vi "Main.vi"() -> ()   [LabVIEW 2021]
doc: "The myRIO Project template acquires acceleration data from the onboard accelerometer and displays the changes of acceleration values in a waveform chart."
uses:
  <vilib>/myRIO/Instrument Drivers/Onboard IO/I2C/typedefs/I2C User Configuration.ctl
  <vilib>/myRIO/Instrument Drivers/Onboard IO/I2C/typedefs/I2C Transfer Rate.ctl
  <vilib>/Platform/TimedLoop/XDataNode/timing_clust.ctl
  <vilib>/Platform/TimedLoop/XDataNode/nitl_modes.ctl
  <vilib>/Platform/TimedLoop/XDataNode/wakeup.ctl
  <vilib>/myRIO/Common/Instrument Driver Framework/myRIO v1.0/UART/vis/myRIO v1.0 Close UART.vi
  <vilib>/Utility/error.llb/Error Cluster From Error Code.vi
  <vilib>/myRIO/Common/Instrument Driver Framework/myRIO v1.0/I2C/vis/myRIO v1.0 Configure I2C.vi
  <vilib>/myRIO/Common/Instrument Driver Framework/myRIO v1.0/DIO/vis/myRIO v1.0 Read DIO.vi
  <vilib>/myRIO/Common/Instrument Driver Framework/myRIO v1.0/I2C/vis/myRIO v1.0 Write I2C.vi
  <vilib>/myRIO/Common/Instrument Driver Framework/myRIO v1.0/AI/vis/myRIO v1.0 Read AI.vi
  <vilib>/express/express analysis/Spectral/Block/exnSpectralBlock spectral measurements power poly.vi
  <vilib>/express/express analysis/Spectral/Block/exnSpectralBlock spectral measurements power DDT.vi
  <vilib>/myRIO/Common/Instrument Driver Framework/Utilities/vis/FPGA Ref Manager.vi
  <vilib>/myRIO/Common/Instrument Driver Framework/myRIO v1.0/myRIO v1.0 Reset FPGA.vi
  <vilib>/myRIO/Common/Instrument Driver Framework/myRIO v1.0/IRQ/vis/myRIO v1.0 IRQ Info FGV.vi
  <vilib>/myRIO/Common/Instrument Driver Framework/myRIO v1.0/IRQ/vis/myRIO v1.0 Timer IRQ Info FGV.vi
  <vilib>/myRIO/Common/Instrument Driver Framework/myRIO v1.0/IRQ/vis/myRIO v1.0 ISR Agent.vi
  <vilib>/myRIO/Instrument Drivers/Utilities/vis/Reset Index.vi
  <vilib>/myRIO/Common/Instrument Driver Framework/myRIO v1.0/Resource Manager/vis/myRIO v1.0 Block Write Resource Manager.vi
  <vilib>/Platform/TimedLoop/XDataNode/XDataNode.xnode
  <vilib>/express/express analysis/Spectral/XNode/ExpressSpectralMeasurementsBlockNode.xnode
  <vilib>/Platform/TimedLoop/XDataNode/XDNodeRunTimeDep.lvlib
  <vilib>/myRIO/Instrument Drivers/Onboard IO/AI/AI.lvlib
  <vilib>/myRIO/Instrument Drivers/Onboard IO/DIO/DIO.lvlib
  <vilib>/Analysis/NI_AAL_SigProc.lvlib
  <vilib>/Analysis/NI_AALPro.lvlib
  <vilib>/myRIO/Instrument Drivers/Utilities/Utilities.lvlib
  <vilib>/myRIO/Instrument Drivers/Onboard IO/I2C/I2C.lvlib
panel:
  in  "Stop Button 2":bool
  in  "Tab Control":T1(tab)
  out "SpO2 (%)":dbl
  in  "Collect Data 3":bool
  in  "R Offset":dbl=0.6
  in  "IR Offset":dbl=0.24
  in  "% Threshold":dbl=0.5 format="%0.2f"
  in  "Width":i32=20 min=3
  out "Heart Rate (bpm)":i32
  out "Filtered Readings 2":dynamicdata(graph)
  out "Frequency Analysis Power Spectrum":dynamicdata(graph)
  in  "Period (> 3s)":dbl=10.0
  in  "Interval (ms)":i64=1
  in  "[ESC] 3":bool
  out "LCD display":string
  out "Imax R":dbl
  out "Imin R":dbl
  out "Imax IR":dbl
  out "Imin IR":dbl
  out "Max Freq R":dbl
  out "Max Freq IR":dbl
  in  "dt (ms)":i64=1
  out "Vpp R":dbl format="%.2p"
  out "Vpp IR":dbl format="%.2p"
  in  "Period (s)":dbl=10.0
  in  "Collect Data 2":bool
  out "Power Spectrum":dynamicdata(graph)
  out "Filtered Readings":dynamicdata(graph)
  out "Heart Rate (bpm)":i32
  in  "width":i32=20 min=3
  in  "threshold":dbl=0.002 format="%0.4f"
  in  "R Offset":dbl
  in  "IR Offset":dbl
  out "Channel Readings":T2(graph)
  in  "[ESC] 2":bool
  out "Blood Oxygen Saturation":dbl
  in  "Absorbance Ratio (R / IR)":dbl(slide) scale=0.0..1.0
  in  "Use Direct Input":bool
  out "LCD display":string
  in  "[ESC]":bool
  in  "Blood Oxygen Input":dbl
  in  "Heart Rate":i32
  in  "Display Data":bool
  in  "eHb, lam1":dbl=0.81
  in  "eHb, lam2":dbl=0.18
  in  "eHbO2, lam1":dbl=0.08
  in  "eHbO2, lam2":dbl=0.29
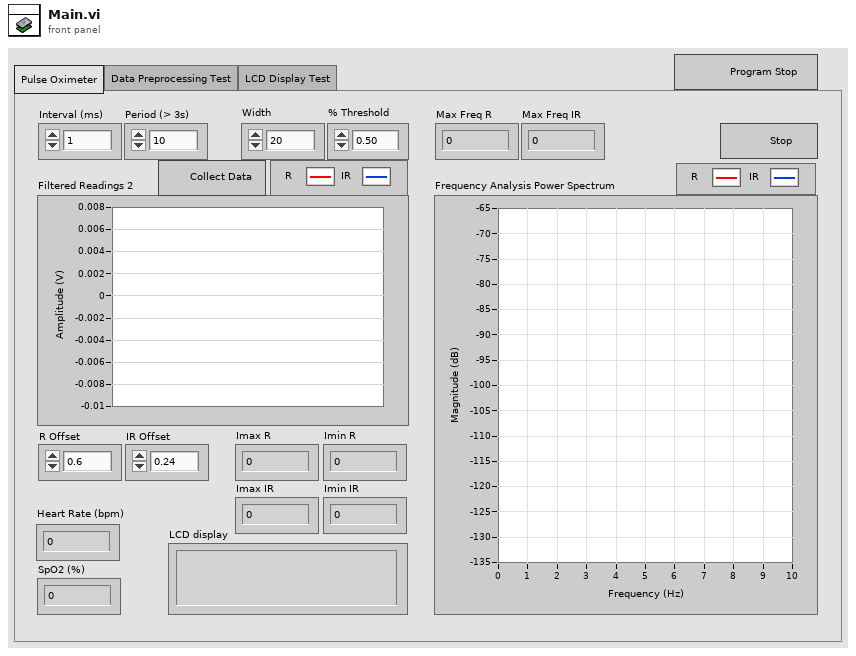
[diagram p1: front panel]
types:
  T1 = enum32{"Pulse Oximeter", "Data Preprocessing Test", "LCD Display Test", "Custom Graphs"}
  T2 = cluster{"dbl Scaled Value":dbl, "dbl Scaled Value":dbl}
  T3 = typedef "I2C.lvlib/I2C User Configuration.ctl" = cluster{"I2C Transfer Rate":T4}
  T4 = typedef "I2C.lvlib/I2C Transfer Rate.ctl" = enum16{"Standard mode (100 kbps)", "Fast mode (400 kbps)"}
  T5 = typedef "I2C.lvlib/I2C Reference.ctl" = cluster{"myRIO Reference":T6, "I2C Channels Enum":T10, "I2C Configuration":T11}
  T6 = typedef "myRIO Generic Hardware Reference.ctl" = cluster{"myRIO Model":T7, "myRIO Hardware Reference":T8}
  T7 = typedef "Hardware Version Enum.ctl" = enum16{"Unknown", "myRIO-1900", "myRIO-1950", "roboRIO", "NI ELVIS RIO CM", "ELVIS III"}
  T8 = typedef "myRIO v1.0 Reference.ctl" = cluster{"Generic FPGA Reference":T9, "Allow multiple opens":bool}
  T9 = typedef "Generic FPGA Reference.ctl" = refnum<k20>
  T10 = typedef "I2C Channels Enum.ctl" = enum16{"Not Connected", "A/I2C", "B/I2C", "I2C/I2C"}
  T11 = typedef "I2C.lvlib/I2C Configuration.ctl" = cluster{"I2C Transfer Rate":T4}
  T12 = typedef "DIO.lvlib/DIO Reference.ctl" = cluster{"myRIO Reference":T6, "DIO Channels List":T13}
  T13 = typedef "DIO Channels List.ctl" = T14[]
  T14 = typedef "DIO Channels Enum.ctl" = enum16{"Not Connected", "C/DIO0", "C/DIO1", "C/DIO2", "C/DIO3", "C/DIO4", "C/DIO5", "C/DIO6", "C/DIO7", "A/DIO0", "A/DIO1", "A/DIO2", "A/DIO3", "A/DIO4", "A/DIO5", "A/DIO6", "A/DIO7", "A/DIO8", "A/DIO9", "A/DIO10", "A/DIO11", "A/DIO12", "A/DIO13", "A/DIO14", "A/DIO15", "A/DIO16", "A/DIO17", "A/DIO18", "A/DIO19", "B/DIO0", "B/DIO1", "B/DIO2", "B/DIO3", "B/DIO4", "B/DIO5", "B/DIO6", "B/DIO7", "B/DIO8", "B/DIO9", "B/DIO10", "B/DIO11", "B/DIO12", "B/DIO13", "B/DIO14", "B/DIO15", "B/DIO16", "B/DIO17", "B/DIO18", "B/DIO19", "LED0", "LED1", "LED2", "LED3", "Button0", "DIO/DIO0", "DIO/DIO1", "DIO/DIO2", "DIO/DIO3", "DIO/DIO4", "DIO/DIO5", "DIO/DIO6", "DIO/DIO7", "DIO/DIO8", "DIO/DIO9", "SPI/CS0", "SPI/CS1", "SPI/CS2", "SPI/CS3", "LED RADIO (Green)", "LED RADIO (Red)", "LED COMM (Green)", "LED COMM (Red)", "LED MODE (Green)", "LED MODE (Red)"}
  T15 = typedef "AI.lvlib/AI Reference.ctl" = cluster{"myRIO Reference":T6, "AI Channels List":T16, "AI Scaling Constants List":T18}
  T16 = typedef "AI Channels List.ctl" = T17[]
  T17 = typedef "AI Channels Enum.ctl" = enum16{"Not Connected", "AudioIn/Left", "AudioIn/Right", "C/AI0", "C/AI1", "A/AI0", "A/AI1", "A/AI2", "A/AI3", "A/AI4", "A/AI5", "A/AI6", "A/AI7", "B/AI0", "B/AI1", "B/AI2", "B/AI3", "B/AI4", "B/AI5", "B/AI6", "B/AI7", "AI/AI0", "AI/AI1", "AI/AI2", "AI/AI3", "A/AI0 (DIFF)", "A/AI1 (DIFF)", "A/AI2 (DIFF)", "A/AI3 (DIFF)", "B/AI0 (DIFF)", "B/AI1 (DIFF)", "B/AI2 (DIFF)", "B/AI3 (DIFF)"}
  T18 = typedef "Analog Scaling Constants List.ctl" = T19[]
  T19 = typedef "Analog Scaling Constants.ctl" = cluster{"LSB Weight (Volts)":dbl, "Offset (Volts)":dbl, "Signed?":bool}
  T20 = typedef "XDNodeRunTimeDep.lvlib/timing_clust.ctl" = cluster{"Expected End [f-1]":u64, "Actual End [f-1]":u64, "Finished Late? [f-1]":bool, "Expected End [i-1]":u64, "Actual End [i-1]":u64, "Finished Late? [i-1]":bool, "Expected Start [i]":u64, "Actual Start [i]":u64, "Expected Start [f]":u64, "Actual Start [f]":u64, "Source Name":string, "Structure Name":string, "Period":i64, "Deadline":i64, "Offset":i64, "Start":i64, "Priority":i32, "Timeout":i32, "Mode":T21, "Wakeup Reason":T22, "Error":errorcluster, "Source Type":string, "Secondary Source Type":string, "Global End Time":u64, "Global Start Time":u64, "Frame Duration":u64, "Iteration Duration":u64, "Assigned CPU":i32, "I/O Scan Engine Mode":u32}
  T21 = typedef "XDNodeRunTimeDep.lvlib/nitl_modes.ctl" = enum32{"No Change", "Process missed periods, maintain original phase", "Discard missed periods, maintain original phase", "Process missed periods, ignore original phase", "Discard missed periods, ignore original phase"}
  T22 = typedef "XDNodeRunTimeDep.lvlib/wakeup.ctl" = enum32{"Normal", "Aborted", "Asynchronous wakeup", "Timing source error", "Timed loop error", "Timeout"}
  T23 = cluster{"averaging mode":u16, "weighting mode":u16, "number of averages":u32}
  T24 = cluster{"dB On (F)":bool, "unwrap phase (F)":bool, "convert to degree (F)":bool}
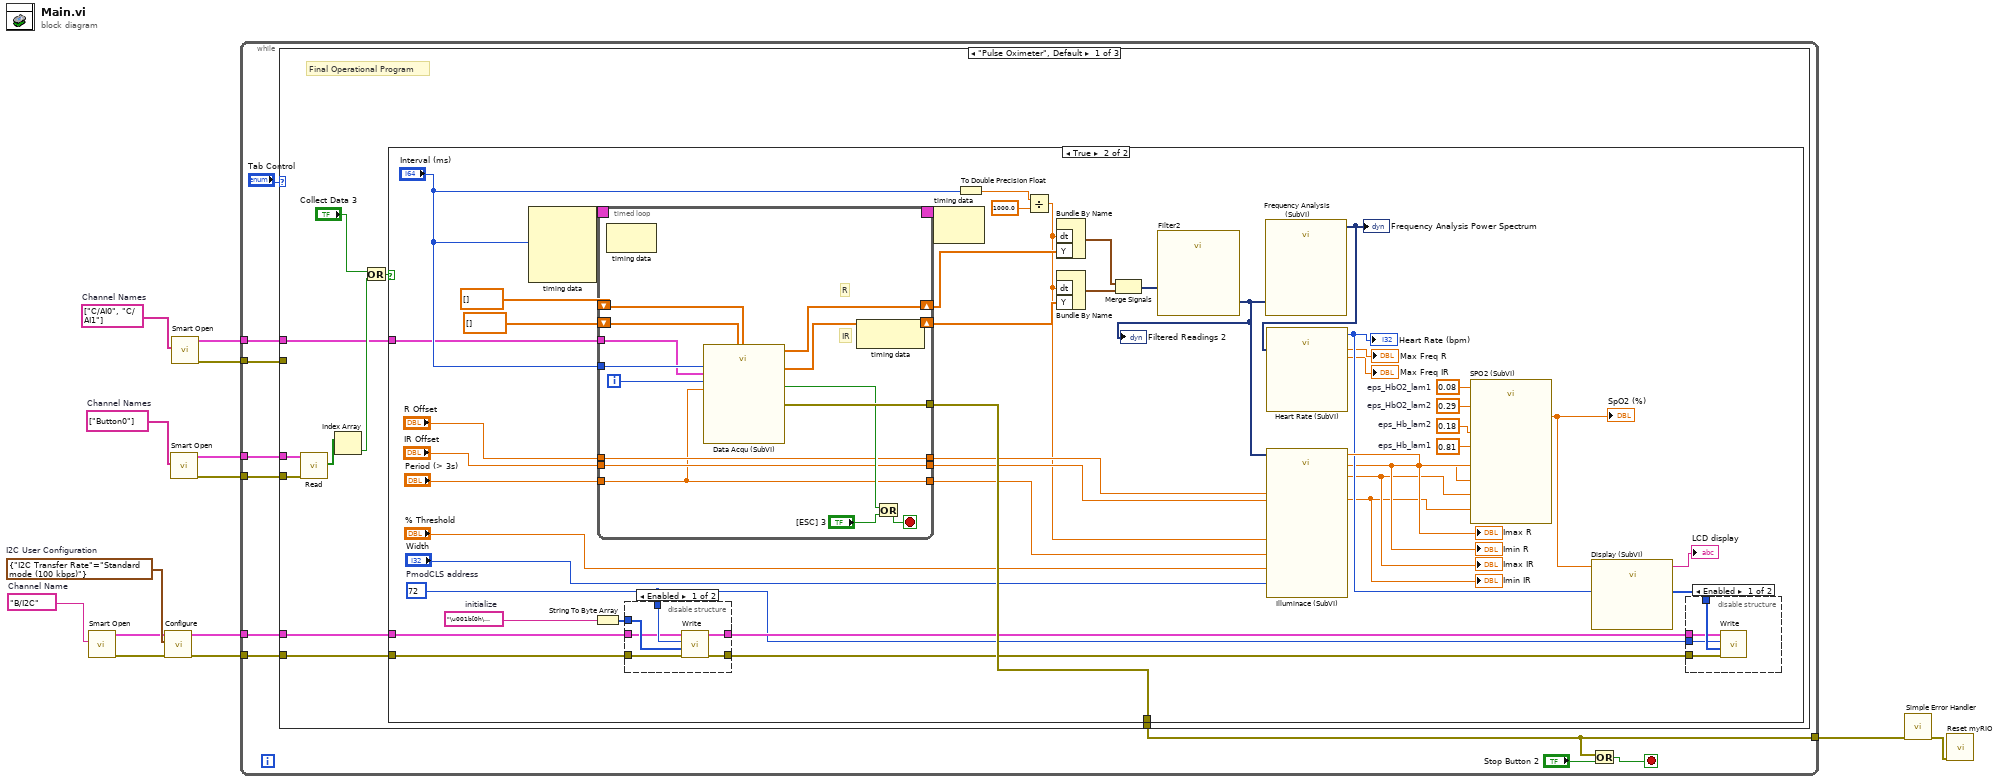
[diagram p0: block diagram]
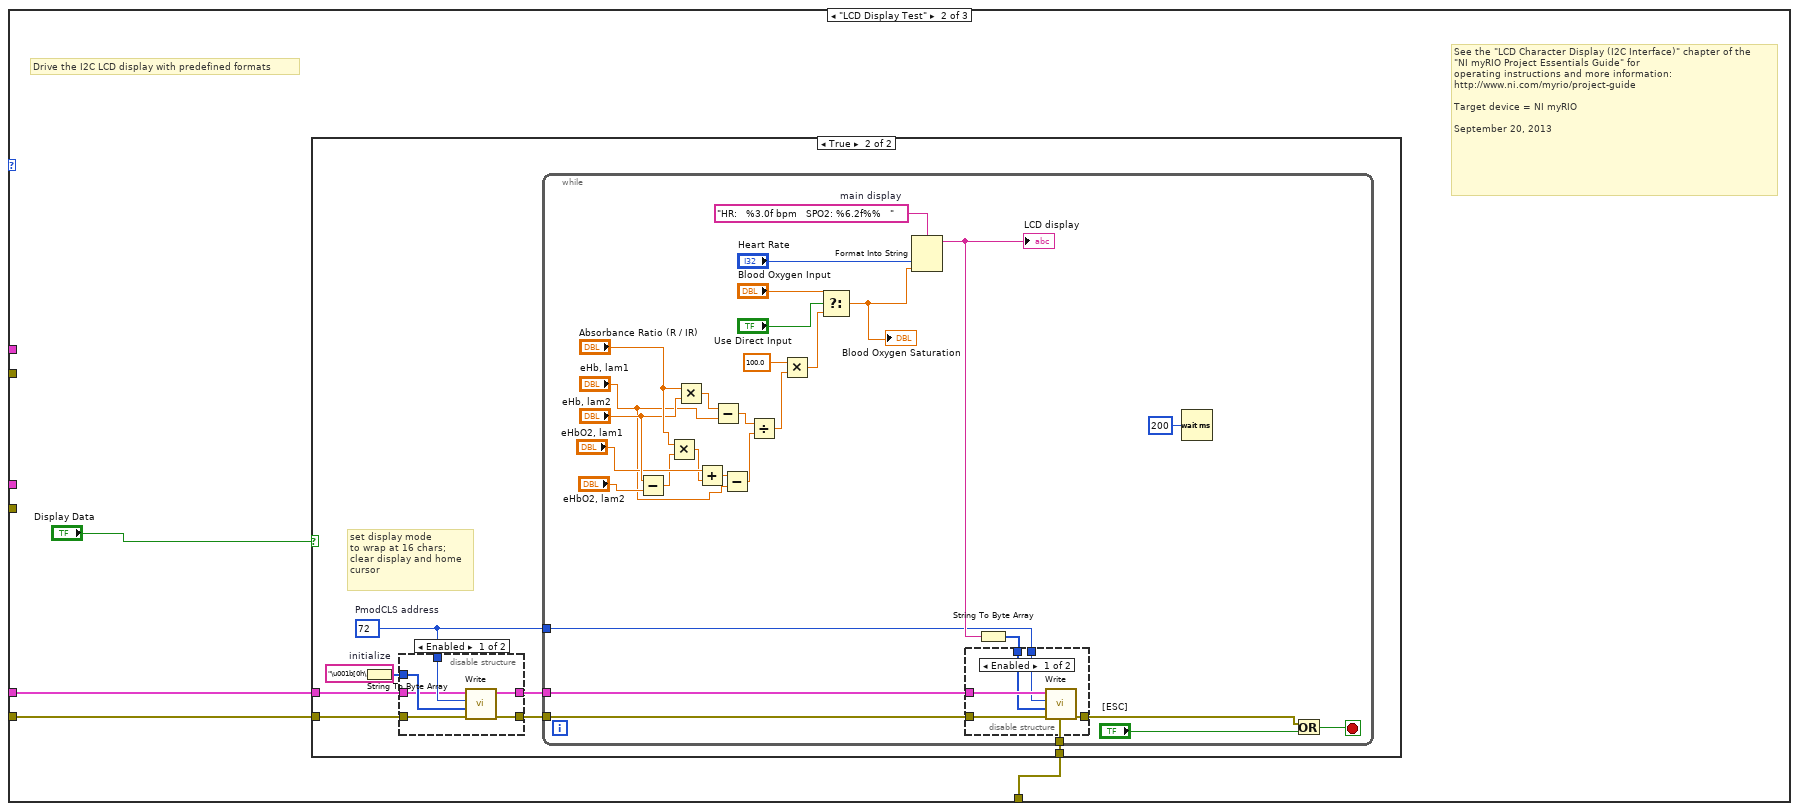
[diagram p5: hidden frame]
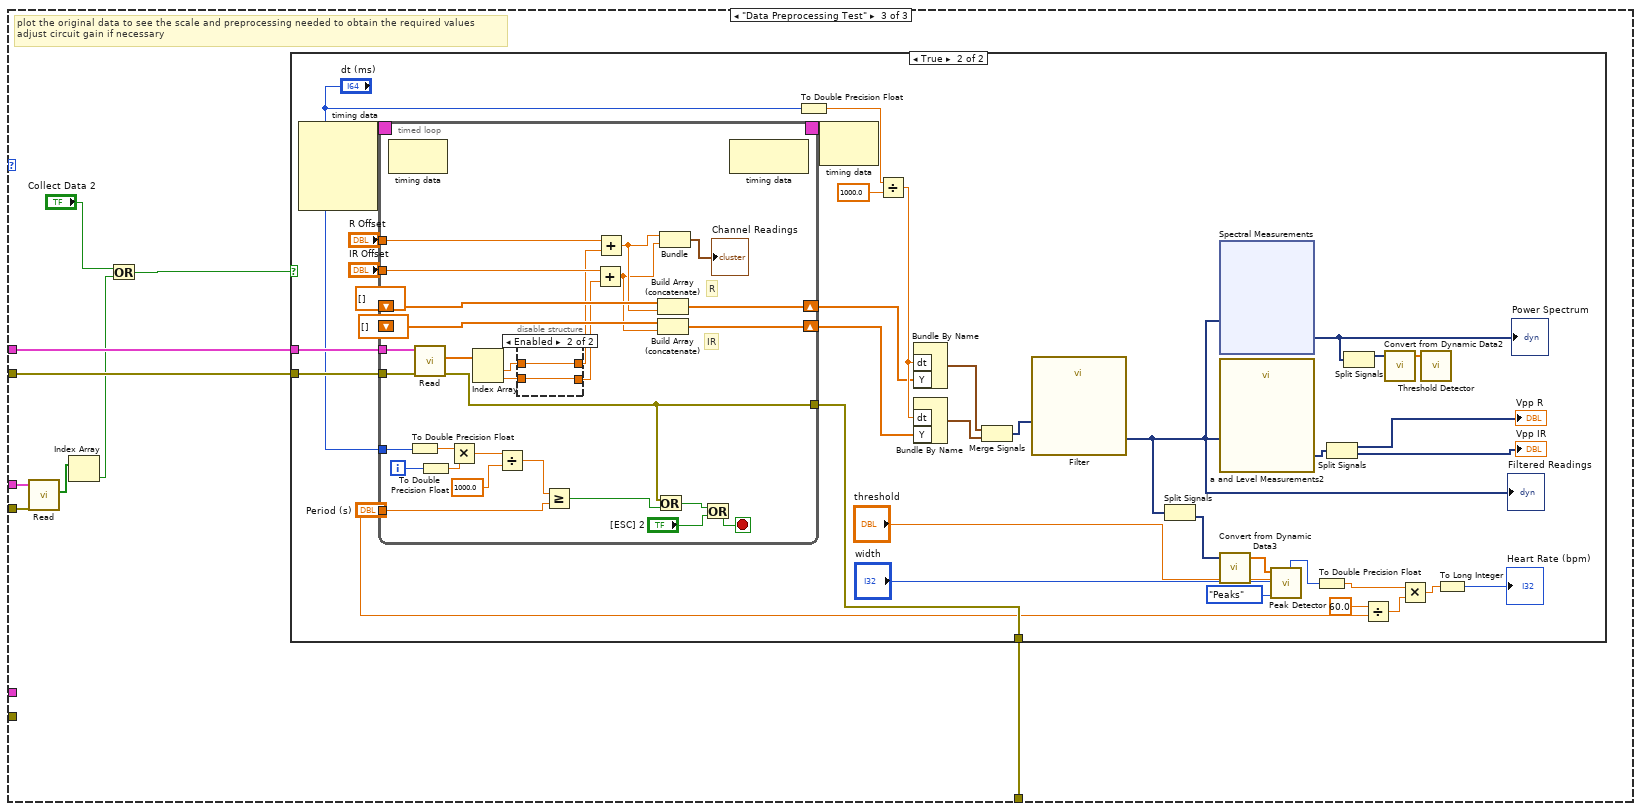
[diagram p9: hidden frame]
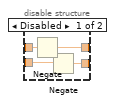
[diagram p11: hidden frame]
diagram:
  w5 = T3 {"I2C Transfer Rate"=enum."Standard mode (100 kbps)"}  # I2C User Configuration
  w6 = tag "B/I2C"  # Channel Name
  w11 = tag[] ["Button0"]  # Channel Names
  w14 = tag[] ["C/AI0", "C/AI1"]  # Channel Names
  n1 = call <vilib>:"Smart Open.vi"("Channel Name"=w6) -> ("error out"=w3:errorcluster, "I2C Ref Out"=w4:T5)  [unwired: 9 in]
  n2 = call <vilib>:"Configure.vi"("error in (no error)"=w3, "I2C User Configuration"=w5, "I2C Ref In"=w4) -> ("error out"=w2:errorcluster, "I2C Ref Out"=w1:T5)  [unwired: 7 in]
  n3 = call <vilib>:"Smart Open.vi"("Channel Names"=w11) -> ("error out"=w9:errorcluster, "DIO Ref Out"=w10:T12)  [unwired: 9 in]
  n4 = call <vilib>:"Smart Open.vi"("Channel Names"=w14) -> ("error out"=w12:errorcluster, "AI Ref Out"=w13:T15)  [unwired: 9 in]
  n5 = while {
    tunnel: w13 -> [w24]
    tunnel: w12 -> [w23]
    tunnel: w10 -> [w21]
    tunnel: w9 -> [w20]
    tunnel: [w17] -> w7
    tunnel: w2 -> [w15]
    tunnel: w1 -> [w16]
    stop <- w18 stop-if-true
    n6 = case shown="\"Pulse Oximeter\", Default" "Tab Control" {
      tunnel: w24 -> [w27 _ w176]
      tunnel: w23 -> [_ _ w175]
      tunnel: w21 -> [w31 _ w174]
      tunnel: w20 -> [w30 _ w173]
      tunnel: [w28 w117 w168] -> w17
      tunnel: w16 -> [w26 w115 _]
      tunnel: w15 -> [w25 w114 _]
      frame "Pulse Oximeter", Default {
        # "Final Operational Program"
        n7 = call <vilib>:"Read.vi"("error in (no error)"=w30, "DIO Ref In"=w31) -> ("Values"=w34:bool[])  [unwired: 7 in, 2 out]
        n8 = Index Array(array=w34) -> (element=w32:bool)  [unwired: 1 in]
        n9 = Or(x="Collect Data 3", y=w32) -> (x .or. y?=w29:bool)
        n10 = case shown="True" w29 {
          tunnel: [_ w68] -> w28
          tunnel: w27 -> [_ w62]
          tunnel: w26 -> [_ w45]
          tunnel: w25 -> [_ w44]
          frame False {
          }
          frame True {
            w46 = u8 72  # PmodCLS address
            w50 = "\u001b[0h\u001b[j"  # initialize
            w63 = 0.81  # eps_Hb_lam1
            w65 = 0.29  # eps_HbO2_lam2
            w67 = 0.08  # eps_HbO2_lam1
            w64 = 0.18  # eps_Hb_lam2
            n11 = node-c288("Interval (ms)") -> (w80:T20)  [unwired: 3 in]
            n12 = String To Byte Array(string=w50) -> (unsigned byte array=w49:u8[])
            n13 = timed-loop {
              timing: w80 -> [_]
              timing-out: [_] -> w79
              shift-right: [w94] -> w40
              shift-left: dbl[] [] -> [w93]
              shift-right: [w92] -> w39
              shift-left: dbl[] [] -> [w91]
              tunnel: "Interval (ms)" -> [w85]
              tunnel: "Period (> 3s)" -> [w81]
              tunnel: "R Offset" -> [w82]
              tunnel: "IR Offset" -> [w83]
              tunnel: [w89] -> w68
              tunnel: w62 -> [w84]
              tunnel: [w83] -> w37
              tunnel: [w82] -> w38
              tunnel: [w81] -> w35
              i -> [w90]
              stop <- w88 stop-if-true
              # "IR"
              # "R"
              n14 = node-c288() -> ()  [unwired: 1 in, 1 out]
              n15 = call "Data Acqu (SubVI).vi"("Period (s) in"=w81, "Numeric"=w90, "AI Ref In"=w84, "dt (ms) in"=w85, "Array in"=w91, "Array 3"=w93) -> ("error out"=w89:errorcluster, "Boolean"=w87:bool, "Array out"=w92:dbl[], "Array 4"=w94:dbl[])  [unwired: 2 in]
              n16 = node-c288() -> ()  [unwired: 1 in, 1 out]
              n17 = Or(x=w87, y="[ESC] 3") -> (x .or. y?=w88:bool)
            }
            n18 = disable-structure shown="Enabled" {
              disable-tunnel: w46 -> [w105 _]
              disable-tunnel: w44 -> [w100 w106]
              disable-tunnel: w49 -> [w104 _]
              disable-tunnel: w45 -> [w101 w107]
              disable-tunnel: [w103 w106] -> w47
              disable-tunnel: [w102 w107] -> w48
              frame Enabled {
                n19 = call <vilib>:"Write.vi"("error in (no error)"=w100, "Bytes to Write"=w104, "Slave Address (7-bit)"=w105, "I2C Ref In"=w101) -> ("error out"=w103:errorcluster, "I2C Ref Out"=w102:T5)  [unwired: 6 in]
              }
              frame Disabled {
              }
            }
            n20 = node-c288(w79) -> ()  [unwired: 1 out]
            n21 = To Double Precision Float(number="Interval (ms)") -> (double precision float=w77:dbl)
            n22 = Divide(x=w77, y=1000.0) -> (x/y=w36:dbl)
            n23 = Bundle By Name("dt"=w36, "Y"=w40) -> (w74:waveform(dbl))  [unwired: 1 in]
            n24 = Bundle By Name("dt"=w36, "Y"=w39) -> (w73:waveform(dbl))  [unwired: 1 in]
            n25 = Merge Signals(w74, w73) -> (w72:dynamicdata)
            n26 = call "Filter2"("Signal"=w72) -> ("Filtered Signal"=w61:dynamicdata)  [unwired: 9 in, 1 out]
            "Filtered Readings 2" <- w61
            n27 = call "Frequency Analysis (SubVI).vi"("Filtered Signal"=w61) -> ("Power Spectrum"=w41:dynamicdata)  [unwired: 8 in, 2 out]
            "Frequency Analysis Power Spectrum" <- w41
            n28 = call "Heart Rate (SubVI).vi"("Power Spectrum"=w41) -> ("Max Freq IR"=→"Max Freq IR":dbl, "Max Freq R"=→"Max Freq R":dbl, "Avg HR bpm"=w56:i32)  [unwired: 7 in, 1 out]
            "Heart Rate (bpm)" <- w56
            n29 = call "Illuminace (SubVI).vi"("R Offset"=w38, "Interval"=w36, "IR Offset"=w37, "Period (> 3s)"=w35, "Width"="Width", "% Threshold"="% Threshold", "Filtered Signal"=w61) -> ("Imax IR"=w53:dbl, "Imin R"=w54:dbl, "Imax R"=w58:dbl, "Imin IR"=w52:dbl)  [unwired: 1 out]
            "Imax R" <- w58
            "Imin R" <- w54
            "Imax IR" <- w53
            "Imin IR" <- w52
            n30 = call "SPO2 (SubVI).vi"("I_max_lam1"=w58, "eps_Hb_lam2"=w64, "I_min_lam2"=w52, "eps_Hb_lam1"=w63, "I_max_lam2"=w53, "eps_HbO2_lam2"=w65, "I_min_lam1"=w54, "eps_HbO2_lam1"=w67) -> ("Numeric"=w55:dbl)  [unwired: 3 in]
            "SpO2 (%)" <- w55
            n31 = call "Display (SubVI).vi"("Numeric 2"=w56, "Numeric"=w55) -> ("Formatted Array"=w51:u8[], "Formatted String"=→"LCD display":string)  [unwired: 8 in]
            n32 = disable-structure shown="Enabled" {
              disable-tunnel: w47 -> [w108 w112]
              disable-tunnel: w51 -> [w111 _]
              disable-tunnel: w46 -> [w110 _]
              disable-tunnel: w48 -> [w109 _]
              frame Enabled {
                n33 = call <vilib>:"Write.vi"("error in (no error)"=w108, "Bytes to Write"=w111, "Slave Address (7-bit)"=w110, "I2C Ref In"=w109) -> ()  [unwired: 6 in, 2 out]
              }
              frame Disabled {
              }
            }
          }
        }
      }
      frame "LCD Display Test" {
        # "See the \"LCD Character Display (I2C Interface)\" chapter of the\n\"NI myRIO Project Essentials Guide\" for\noperating instructions and more information: \nhttp://www.ni.com/myrio/project-guide\n\nTarget device = NI myRIO\n\nSeptember 20, 2013"
        # "Drive the I2C LCD display with predefined formats"
        n34 = case shown="True" "Display Data" {
          tunnel: [_ w124] -> w117
          tunnel: w115 -> [_ w119]
          tunnel: w114 -> [_ w118]
          frame False {
          }
          frame True {
            w123 = u8 72  # PmodCLS address
            w125 = "\u001b[0h\u001b[j"  # initialize
            # "set display mode\nto wrap at 16 chars;\nclear display and home\ncursor"
            n35 = String To Byte Array(string=w125) -> (unsigned byte array=w122:u8[])
            n36 = disable-structure shown="Enabled" {
              disable-tunnel: w123 -> [w131 _]
              disable-tunnel: w118 -> [w126 w132]
              disable-tunnel: w122 -> [w130 _]
              disable-tunnel: w119 -> [w127 w133]
              disable-tunnel: [w129 w132] -> w121
              disable-tunnel: [w128 w133] -> w120
              frame Enabled {
                n37 = call <vilib>:"Write.vi"("error in (no error)"=w126, "Bytes to Write"=w130, "Slave Address (7-bit)"=w131, "I2C Ref In"=w127) -> ("error out"=w129:errorcluster, "I2C Ref Out"=w128:T5)  [unwired: 6 in]
              }
              frame Disabled {
              }
            }
            n38 = while {
              tunnel: w123 -> [w152]
              tunnel: [w155] -> w124
              tunnel: w121 -> [w156]
              tunnel: w120 -> [w154]
              stop <- w159 stop-if-true
              w161 = "HR:   %3.0f bpm   SPO2: %6.2f%%   "  # main display
              n39 = Subtract(x="eHb, lam2", y="eHbO2, lam2") -> (x-y=w140:dbl)
              n40 = Multiply(x="Absorbance Ratio (R / IR)", y=w140) -> (x*y=w139:dbl)
              n41 = Multiply(x="Absorbance Ratio (R / IR)", y="eHb, lam2") -> (x*y=w148:dbl)
              n42 = Add(x="eHbO2, lam1", y=w139) -> (x+y=w142:dbl)
              n43 = Subtract(x=w148, y="eHb, lam1") -> (x-y=w147:dbl)
              n44 = Subtract(x=w142, y="eHb, lam1") -> (x-y=w138:dbl)
              n45 = Divide(x=w147, y=w138) -> (x/y=w137:dbl)
              n46 = Multiply(x=100.0, y=w137) -> (x*y=w135:dbl)
              n47 = Select(t="Blood Oxygen Input", s="Use Direct Input", f=w135) -> (s? t:f=w134:dbl)
              "Blood Oxygen Saturation" <- w134
              n48 = Format Into String "Format Into String"(format string=w161, "Heart Rate", w134) -> (resulting string=w157:string)  [unwired: 2 in, 1 out]
              "LCD display" <- w157
              n49 = String To Byte Array(string=w157) -> (unsigned byte array=w153:u8[])
              n50 = disable-structure shown="Enabled" {
                disable-tunnel: w156 -> [w166 w167]
                disable-tunnel: [w165 w167] -> w155
                disable-tunnel: w154 -> [w164 _]
                disable-tunnel: w153 -> [w163 _]
                disable-tunnel: w152 -> [w162 _]
                frame Enabled {
                  n51 = call <vilib>:"Write.vi"("error in (no error)"=w166, "Bytes to Write"=w163, "Slave Address (7-bit)"=w162, "I2C Ref In"=w164) -> ("error out"=w165:errorcluster)  [unwired: 6 in, 1 out]
                }
                frame Disabled {
                }
              }
              n52 = Wait (ms)(milliseconds to wait=u32 200) -> ()  [unwired: 1 out]
              n53 = Or(x=w155, y="[ESC]") -> (x .or. y?=w159:bool)
            }
          }
        }
      }
      frame "Data Preprocessing Test" {
        # "plot the original data to see the scale and preprocessing needed to obtain the required values\nadjust circuit gain if necessary"
        n54 = call <vilib>:"Read.vi"("error in (no error)"=w173, "DIO Ref In"=w174) -> ("Values"=w172:bool[])  [unwired: 7 in, 2 out]
        n55 = Index Array(array=w172) -> (element=w169:bool)  [unwired: 1 in]
        n56 = Or(x="Collect Data 2", y=w169) -> (x .or. y?=w170:bool)
        n57 = case shown="True" w170 {
          tunnel: w176 -> [_ w211]
          tunnel: w175 -> [_ w210]
          tunnel: [_ w181] -> w168
          frame False {
          }
          frame True {
            n58 = node-c288("dt (ms)") -> (w213:T20)  [unwired: 3 in]
            n59 = timed-loop {
              timing: w213 -> [_]
              timing-out: [_] -> w212
              tunnel: w211 -> [w242]
              tunnel: w210 -> [w241]
              shift-right: [w240] -> w205
              shift-left: dbl[] [] -> [w239]
              shift-right: [w238] -> w204
              shift-left: dbl[] [] -> [w237]
              tunnel: "dt (ms)" -> [w232]
              tunnel: "Period (s)" -> [w229]
              tunnel: "R Offset" -> [w227]
              tunnel: "IR Offset" -> [w226]
              tunnel: [w221] -> w181
              i -> [w234]
              stop <- w220 stop-if-true
              # "IR"
              # "R"
              n60 = node-c288() -> ()  [unwired: 1 in, 1 out]
              n61 = To Double Precision Float(number=w232) -> (double precision float=w231:dbl)
              n62 = call <vilib>:"Read.vi"("error in (no error)"=w241, "AI Ref In"=w242) -> ("error out"=w221:errorcluster, "Values"=w228:dbl[])  [unwired: 7 in, 1 out]
              n63 = To Double Precision Float(number=w234) -> (double precision float=w233:dbl)
              n64 = Multiply(x=w231, y=w233) -> (x*y=w236:dbl)
              n65 = Index Array(array=w228) -> (element #1=w217:dbl, element #2=w215:dbl)  [unwired: 2 in]
              n66 = Divide(x=w236, y=1000.0) -> (x/y=w230:dbl)
              n67 = disable-structure shown="Enabled" {
                disable-tunnel: w217 -> [w246 w248]
                disable-tunnel: [w245 w248] -> w216
                disable-tunnel: w215 -> [w244 w247]
                disable-tunnel: [w243 w247] -> w214
                frame Disabled {
                  n68 = Negate(x=w246) -> (-x=w245:dbl)
                  n69 = Negate(x=w244) -> (-x=w243:dbl)
                }
                frame Enabled {
                }
              }
              n70 = Greater Or Equal?(x=w230, y=w229) -> (x >= y?=w222:bool)
              n71 = Add(x=w226, y=w214) -> (x+y=w223:dbl)
              n72 = Add(x=w227, y=w216) -> (x+y=w224:dbl)
              n73 = Or(x=w221, y=w222) -> (x .or. y?=w219:bool)
              n74 = Build Array (concatenate)(w239, w224) -> (w240:dbl[])
              n75 = Build Array (concatenate)(w237, w223) -> (w238:dbl[])
              n76 = Bundle(w224, w223) -> (→"Channel Readings":cluster{dbl, dbl})  [unwired: 1 in]
              n77 = Or(x=w219, y="[ESC] 2") -> (x .or. y?=w220:bool)
              n78 = node-c288() -> ()  [unwired: 1 in, 1 out]
            }
            n79 = To Double Precision Float(number="dt (ms)") -> (double precision float=w206:dbl)
            n80 = node-c288(w212) -> ()  [unwired: 1 out]
            n81 = Divide(x=w206, y=1000.0) -> (x/y=w208:dbl)
            n82 = Bundle By Name("dt"=w208, "Y"=w205) -> (w201:waveform(dbl))  [unwired: 1 in]
            n83 = Bundle By Name("dt"=w208, "Y"=w204) -> (w200:waveform(dbl))  [unwired: 1 in]
            n84 = Merge Signals(w201, w200) -> (w199:dynamicdata)
            n85 = call "Filter"("Signal"=w199) -> ("Filtered Signal"=w179:dynamicdata)  [unwired: 9 in, 1 out]
            "Filtered Readings" <- w179
            n86 = Split Signals(w179) -> (w177:dynamicdata)  [unwired: 2 in, 1 out]
            n87 = xnode "Spectral Measurements"("Signals"=w179) -> ("Power Spectrum"=w194:dynamicdata)  [unwired: 1 in, 1 out]
            "Power Spectrum" <- w194
            n88 = call "a and Level Measurements2"("Signals"=w179) -> ("Peak to Peak"=w198:dynamicdata)  [unwired: 12 in, 2 out]
            n89 = call "Convert from Dynamic Data3"("Dynamic Data Type"=w177) -> ("Array"=w195:dbl[])  [unwired: 3 in]
            n90 = call <vilib>:"Peak Detector.vi"("peaks/valleys"=enum32{"Peaks", "Valleys"}."Peaks", "width"="width", "threshold"="threshold", "X"=w195) -> ("# found"=w192:i32)  [unwired: 3 in, 4 out]
            n91 = To Double Precision Float(number=w192) -> (double precision float=w188:dbl)
            n92 = Split Signals(w198) -> (→"Vpp R":dynamicdata, →"Vpp IR":dynamicdata)  [unwired: 2 in]
            n93 = Split Signals(w194) -> (w193:dynamicdata)  [unwired: 2 in, 1 out]
            n94 = Divide(x=60.0, y="Period (s)") -> (x/y=w189:dbl)
            n95 = call "Convert from Dynamic Data2"("Dynamic Data Type"=w193) -> ("Array"=w196:dbl[])  [unwired: 3 in]
            n96 = Multiply(x=w188, y=w189) -> (x*y=w187:dbl)
            n97 = call <vilib>:"Threshold Detector.vi"("X"=w196) -> ()  [unwired: 2 in, 3 out]
            n98 = To Long Integer(number=w187) -> (32bit integer=→"Heart Rate (bpm)":i32)
          }
        }
      }
    }
    n99 = Or(x=w17, y="Stop Button 2") -> (x .or. y?=w18:bool)
  }
  n100 = call <vilib>:"Simple Error Handler.vi"("error in (no error)"=w7) -> ("error out"=w8:errorcluster)  [unwired: 4 in, 4 out]
  n101 = call <vilib>:"Reset myRIO.vi"("error in (no error)"=w8) -> ()  [unwired: 10 in, 1 out]
